vi "VP_AIT 1553 Get BM MonitorData Message At.vi"(7 "error in":errorcluster, 9 "message index in":u32, 10 "monitor data handle in":u32) -> (0 "error out":errorcluster, 2 "VP BM Message":T1[](array[typedef]) {"Data Word array" format="%x"}, 3 "monitor data handle out":u32)   [LabVIEW 2013]
doc: "Returns a summary cluster of the message at a given message index."
uses:
  RT Controls/VP_BM Message.ctl
  <instrlib>/AIT 1553/Private/AIT 1553 Utility/Decode Word/Decode Word (Command as terminals).vi
  <userlib>/MIL-STD-1553/Owl1553.lvlib
  AIT 664 Custom Device.lvlib
  <instrlib>/AIT 1553/AIT 1553.lvlib
panel:
  out "Message We Want":bool
  # "(c) 2010 Avionics Interface Technologies.  ALL RIGHTS RESERVED."
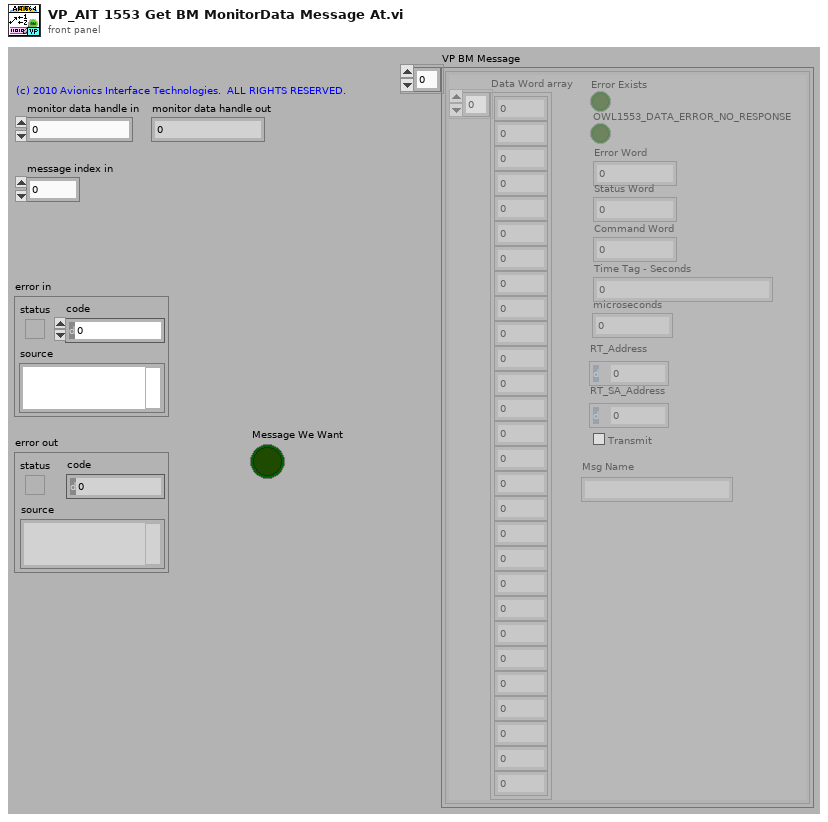
[diagram p1: front panel]
types:
  T1 = typedef "AIT 664 Custom Device.lvlib/VP_BM Message.ctl" = cluster{"Data Word array":u16[], "Error Exists":bool, "OWL1553_DATA_ERROR_NO_RESPONSE":bool, "Error Word":u32, "Status Word":u16, "Command Word":u16, "Time Tag - Seconds":u32, "microseconds":u32, "RT_Address":u8, "RT_SA_Address":u8, "Transmit":bool, "Msg Name":string}
  T2 = enum16{"BCRT", "RTBC", "RTRT", "FRONT_HALF", "BACK_HALF", "MSG_ERROR"}
  T3 = enum16{"OWL1553_BCRT", "OWL1553_RTBC", "OWL1553_RTRT", "OWL1553_FRONT_HALF", "OWL1553_BACK_HALF", "OWL1553_MSG_ERROR"}
  T4 = cluster{"day":u32, "hour":u32, "minute":u32, "second":u32, "microsecond":u32}
  T5 = cluster{"OWL1553_DATA_ERROR_ALTERNATE_BUS":bool, "OWL1553_DATA_ERROR_WORDCOUNT_LOW":bool, "OWL1553_DATA_ERROR_WORDCOUNT_HIGH":bool, "OWL1553_DATA_ERROR_STATUS_WORD":bool, "OWL1553_DATA_ERROR_TERMINAL_ADDRESS":bool, "OWL1553_DATA_ERROR_GAP_SHORT":bool, "OWL1553_DATA_ERROR_ILLEGAL_COMMAND":bool, "OWL1553_DATA_ERROR_BOTH_BUSES":bool, "OWL1553_DATA_ERROR_INTERWORD_GAP":bool, "OWL1553_DATA_ERROR_INVERTED_SYNC":bool, "OWL1553_DATA_ERROR_PARITY":bool, "OWL1553_DATA_ERROR_BITCOUNT_HIGH":bool, "OWL1553_DATA_ERROR_BITCOUNT_LOW":bool, "OWL1553_DATA_ERROR_MANCHESTER":bool, "OWL1553_DATA_ERROR_MANCHESTER_HIGH":bool, "OWL1553_DATA_ERROR_MANCHESTER_LOW":bool, "OWL1553_DATA_ERROR_NO_RESPONSE":bool, "OWL1553_DATA_ERROR_ZERO_CROSSING":bool}
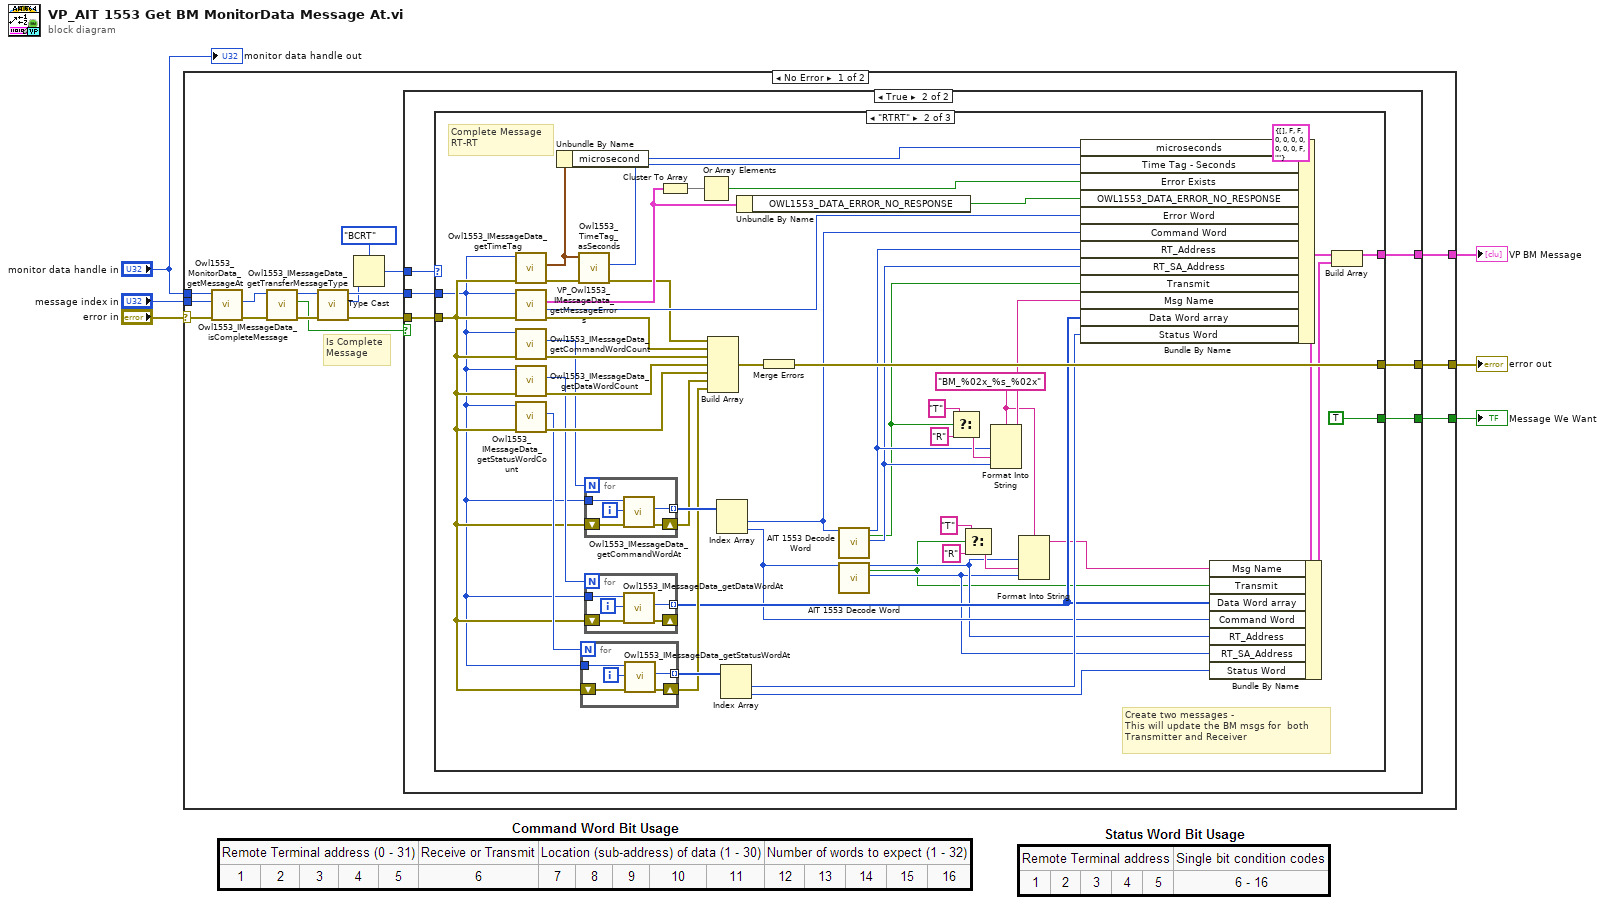
[diagram p0: block diagram]
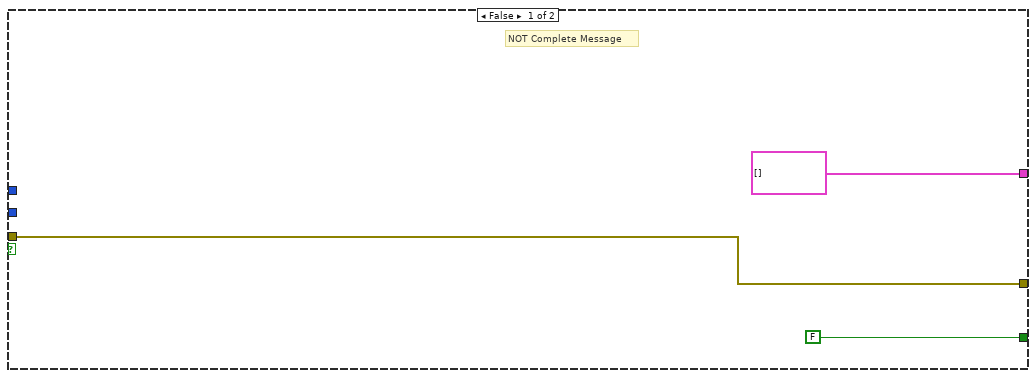
[diagram p2: hidden frame]
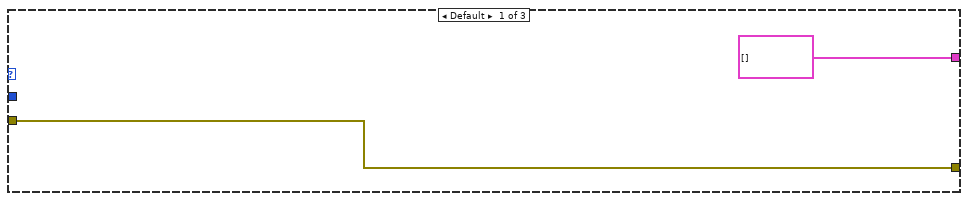
[diagram p3: hidden frame]
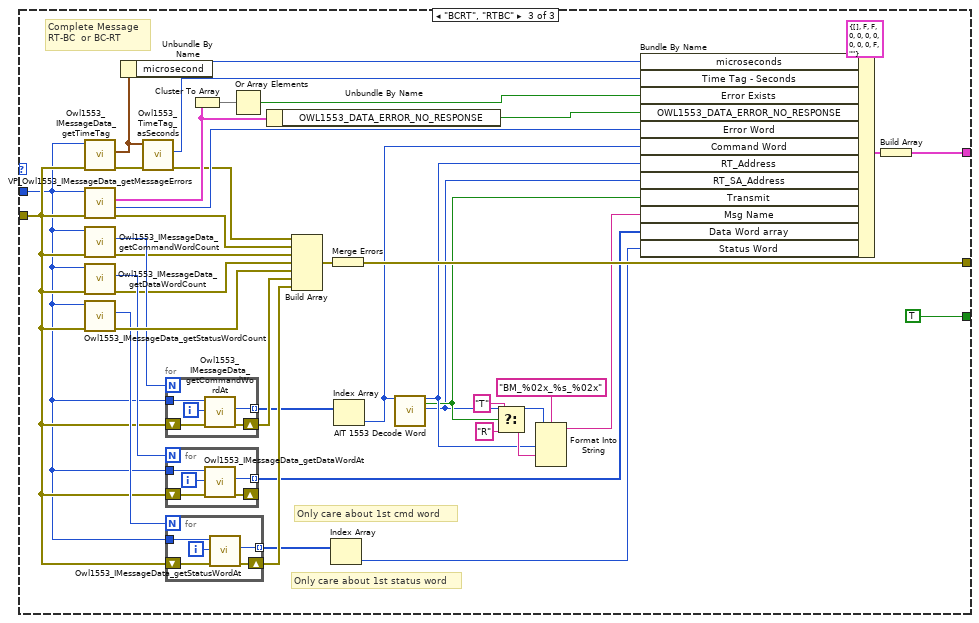
[diagram p4: hidden frame]
diagram:
  n1 = case shown="No Error" "error in" {
    selector: "error in" -> [w21 w154]
    tunnel: [w19 w154] -> w3
    tunnel: "monitor data handle in" -> [w18 _]
    tunnel: "message index in" -> [w22 _]
    tunnel: [w20 _] -> w1
    tunnel: [w9 _] -> w2
    frame No Error {
      # "Is Complete\nMessage"
      n2 = call <userlib>:"Owl1553_MonitorData_getMessageAt.vi"("error in (no error)"=w21, "index"=w22, "monitor data handle"=w18) -> ("error out"=w17:errorcluster, "imessage data handle"=w16:u64)  [unwired: 6 in, 1 out]
      n3 = call <userlib>:"Owl1553_IMessageData_isCompleteMessage.vi"("error in (no error)"=w17, "imessage data handle"=w16) -> ("error out"=w14:errorcluster, "complete"=w8:bool, "imessage data handle"=w15:u64)  [unwired: 7 in]
      n4 = call <userlib>:"Owl1553_IMessageData_getTransferMessageType.vi"("error in (no error)"=w14, "IMessageData handle"=w15) -> ("error out"=w13:errorcluster, "transferMessageType"=w11:T3, "IMessageData handle out"=w12:u64)  [unwired: 7 in]
      n5 = Type Cast(type=T2."BCRT" ("transfer type"), x=w11) -> (*(type *) &x=w7:T2)
      n6 = case shown="True" w8 {
        tunnel: [T1[] [] w31] -> w20
        tunnel: [w24 w30] -> w19
        tunnel: w13 -> [w24 w29]
        tunnel: w12 -> [_ w28]
        tunnel: [FALSE ("Message We Want") w27] -> w9
        tunnel: w7 -> [_ w26]
        frame False {
          # "NOT Complete Message"
        }
        frame True {
          n7 = case shown="\"RTRT\"" w26 {
            tunnel: [T1[] [] w65 w120] -> w31
            tunnel: [w33 w79 w136] -> w30
            tunnel: w29 -> [w33 w68 w123]
            tunnel: w28 -> [_ w67 w122]
            tunnel: [_ TRUE ("Message We Want") TRUE ("Message We Want")] -> w27
            frame Default {
            }
            frame "RTRT" {
              w40 = "BM_%02x_%s_%02x"
              # "Create two messages - \nThis will update the BM msgs for  both\nTransmitter and Receiver"
              # "Complete Message\nRT-RT"
              n8 = call <userlib>:"Owl1553_IMessageData_getTimeTag.vi"("error in (no error)"=w68, "imessage data handle"=w67) -> ("error out"=w74:errorcluster, "time tag"=w71:T4)  [unwired: 7 in, 1 out]
              n9 = call "VP_Owl1553_IMessageData_getMessageErrors.vi"("error in (no error)"=w68, "imessage data handle"=w67) -> ("error out"=w36:errorcluster, "error word"=w69:u32, "DataErrorType"=w57:T5)  [unwired: 6 in, 1 out]
              n10 = call <userlib>:"Owl1553_IMessageData_getCommandWordCount.vi"("error in (no error)"=w68, "imessage data handle"=w67) -> ("error out"=w83:errorcluster, "word count"=w76:u8)  [unwired: 7 in, 1 out]
              n11 = call <userlib>:"Owl1553_IMessageData_getDataWordCount.vi"("error in (no error)"=w68, "imessage data handle"=w67) -> ("error out"=w82:errorcluster, "word count"=w78:u8)  [unwired: 7 in, 1 out]
              n12 = call <userlib>:"Owl1553_IMessageData_getStatusWordCount.vi"("error in (no error)"=w68, "imessage data handle"=w67) -> ("error out"=w81:errorcluster, "word count"=w75:u8)  [unwired: 7 in, 1 out]
              n13 = Unbundle By Name(w71) -> ("microsecond"=w39:u32)
              n14 = call <userlib>:"Owl1553_TimeTag_asSeconds.vi"("error in (no error)"=w74, "time tag"=w71) -> ("error out"=w37:errorcluster, "seconds"=w38:u32)  [unwired: 7 in, 1 out]
              n15 = for {
                N: w75 -> [_]
                shift-right: [w91] -> w53
                shift-left: w68 -> [w92]
                tunnel: w67 -> [w90]
                tunnel: [w89] -> w59 mode=indexing
                i -> [w93]
                n16 = call <userlib>:"Owl1553_IMessageData_getStatusWordAt.vi"("error in (no error)"=w92, "status word index"=w93, "imessage data handle"=w90) -> ("error out"=w91:errorcluster, "word"=w89:u16)  [unwired: 6 in, 1 out]
              }
              n17 = for {
                N: w76 -> [_]
                shift-right: [w86] -> w56
                shift-left: w68 -> [w87]
                tunnel: w67 -> [w85]
                tunnel: [w84] -> w58 mode=indexing
                i -> [w88]
                n18 = call <userlib>:"Owl1553_IMessageData_getCommandWordAt.vi"("error in (no error)"=w87, "command word index"=w88, "imessage data handle"=w85) -> ("error out"=w86:errorcluster, "word"=w84:u16)  [unwired: 6 in, 1 out]
              }
              n19 = for {
                N: w78 -> [_]
                tunnel: w67 -> [w97]
                shift-right: [w94] -> _
                shift-left: w68 -> [w96]
                tunnel: [w95] -> w47 mode=indexing
                i -> [w98]
                n20 = call <userlib>:"Owl1553_IMessageData_getDataWordAt.vi"("error in (no error)"=w96, "data word index"=w98, "imessage data handle"=w97) -> ("error out"=w94:errorcluster, "word"=w95:u16)  [unwired: 6 in, 1 out]
              }
              n21 = Cluster To Array(cluster=w57) -> (array=w77:bool[])
              n22 = Or Array Elements(Boolean array=w77) -> (logical OR=w72:bool)
              n23 = Build Array(w37, w36, w83, w82, w81, w56, w53) -> (w80:errorcluster[])
              n24 = Index Array(array=w58) -> (element #1=w35:u16, element #2=w45:u16)  [unwired: 2 in]
              n25 = Index Array(array=w59) -> (element #1=w54:u16, element #2=w46:u16)  [unwired: 2 in]
              n26 = Unbundle By Name(w57) -> ("OWL1553_DATA_ERROR_NO_RESPONSE"=w70:bool)
              n27 = Merge Errors(w80) -> (w79:errorcluster)
              n28 = call-poly <instrlib>:"AIT 1553 Decode Word.vi"("command word in"=w35) -> ("remote terminal address out"=w61:u16, "transmit out"=w49:bool, "subaddress / mode out"=w60:u16)  [unwired: 15 in, 1 out]
              n29 = call-poly <instrlib>:"AIT 1553 Decode Word.vi"("command word in"=w45) -> ("remote terminal address out"=w44:u16, "transmit out"=w42:bool, "subaddress / mode out"=w43:u16)  [unwired: 15 in, 1 out]
              n30 = Select(t="T", s=w49, f="R") -> (s? t:f=w62:string)
              n31 = Select(t="T", s=w42, f="R") -> (s? t:f=w52:string)
              n32 = Format Into String(format string=w40, w61, w62, w60) -> (resulting string=w55:string)  [unwired: 2 in, 1 out]
              n33 = Format Into String(format string=w40, w44, w52, w43) -> (resulting string=w34:string)  [unwired: 2 in, 1 out]
              n34 = Bundle By Name(cluster=T1 {"Data Word array"=[], "Error Exists"=FALSE, "OWL1553_DATA_ERROR_NO_RESPONSE"=FALSE, "Error Word"=0, "Status Word"=0, "Command Word"=0, "Time Tag - Seconds"=0, "microseconds"=0, "RT_Address"=0, "RT_SA_Address"=0, "Transmit"=FALSE, "Msg Name"=""} ("VP BM Message"), "microseconds"=w39, "Time Tag - Seconds"=w38, "Error Exists"=w72, "OWL1553_DATA_ERROR_NO_RESPONSE"=w70, "Error Word"=w69, "Command Word"=w35, "RT_Address"=w61, "RT_SA_Address"=w60, "Transmit"=w49, "Msg Name"=w55, "Data Word array"=w47, "Status Word"=w54) -> (w48:T1)
              n35 = Bundle By Name(cluster=w48, "Msg Name"=w34, "Transmit"=w42, "Data Word array"=w47, "Command Word"=w45, "RT_Address"=w44, "RT_SA_Address"=w43, "Status Word"=w46) -> (w41:T1)
              n36 = Build Array(w48, w41) -> (w65:T1[])
            }
            frame "BCRT", "RTBC" {
              # "Only care about 1st cmd word"
              # "Only care about 1st status word"
              # "Complete Message\nRT-BC  or BC-RT"
              n37 = call <userlib>:"Owl1553_IMessageData_getTimeTag.vi"("error in (no error)"=w123, "imessage data handle"=w122) -> ("error out"=w129:errorcluster, "time tag"=w126:T4)  [unwired: 7 in, 1 out]
              n38 = call "VP_Owl1553_IMessageData_getMessageErrors.vi"("error in (no error)"=w123, "imessage data handle"=w122) -> ("error out"=w101:errorcluster, "error word"=w104:u32, "DataErrorType"=w125:T5)  [unwired: 6 in, 1 out]
              n39 = call <userlib>:"Owl1553_IMessageData_getCommandWordCount.vi"("error in (no error)"=w123, "imessage data handle"=w122) -> ("error out"=w110:errorcluster, "word count"=w131:u8)  [unwired: 7 in, 1 out]
              n40 = call <userlib>:"Owl1553_IMessageData_getDataWordCount.vi"("error in (no error)"=w123, "imessage data handle"=w122) -> ("error out"=w109:errorcluster, "word count"=w135:u8)  [unwired: 7 in, 1 out]
              n41 = call <userlib>:"Owl1553_IMessageData_getStatusWordCount.vi"("error in (no error)"=w123, "imessage data handle"=w122) -> ("error out"=w138:errorcluster, "word count"=w130:u8)  [unwired: 7 in, 1 out]
              n42 = Unbundle By Name(w126) -> ("microsecond"=w106:u32)
              n43 = call <userlib>:"Owl1553_TimeTag_asSeconds.vi"("error in (no error)"=w129, "time tag"=w126) -> ("error out"=w102:errorcluster, "seconds"=w105:u32)  [unwired: 7 in, 1 out]
              n44 = for {
                N: w131 -> [_]
                shift-right: [w141] -> w133
                shift-left: w123 -> [w142]
                tunnel: w122 -> [w140]
                tunnel: [w139] -> w111 mode=indexing
                i -> [w143]
                n45 = call <userlib>:"Owl1553_IMessageData_getCommandWordAt.vi"("error in (no error)"=w142, "command word index"=w143, "imessage data handle"=w140) -> ("error out"=w141:errorcluster, "word"=w139:u16)  [unwired: 6 in, 1 out]
              }
              n46 = for {
                N: w135 -> [_]
                tunnel: w122 -> [w152]
                shift-right: [w149] -> _
                shift-left: w123 -> [w151]
                tunnel: [w150] -> w107 mode=indexing
                i -> [w153]
                n47 = call <userlib>:"Owl1553_IMessageData_getDataWordAt.vi"("error in (no error)"=w151, "data word index"=w153, "imessage data handle"=w152) -> ("error out"=w149:errorcluster, "word"=w150:u16)  [unwired: 6 in, 1 out]
              }
              n48 = for {
                N: w130 -> [_]
                shift-right: [w146] -> w132
                shift-left: w123 -> [w147]
                tunnel: w122 -> [w145]
                tunnel: [w144] -> w112 mode=indexing
                i -> [w148]
                n49 = call <userlib>:"Owl1553_IMessageData_getStatusWordAt.vi"("error in (no error)"=w147, "status word index"=w148, "imessage data handle"=w145) -> ("error out"=w146:errorcluster, "word"=w144:u16)  [unwired: 6 in, 1 out]
              }
              n50 = Cluster To Array(cluster=w125) -> (array=w134:bool[])
              n51 = Or Array Elements(Boolean array=w134) -> (logical OR=w127:bool)
              n52 = Unbundle By Name(w125) -> ("OWL1553_DATA_ERROR_NO_RESPONSE"=w124:bool)
              n53 = Build Array(w102, w101, w110, w109, w138, w133, w132) -> (w137:errorcluster[])
              n54 = Index Array(array=w112) -> (element=w103:u16)  [unwired: 1 in]
              n55 = Merge Errors(w137) -> (w136:errorcluster)
              n56 = Index Array(array=w111) -> (element=w100:u16)  [unwired: 1 in]
              n57 = call-poly <instrlib>:"AIT 1553 Decode Word.vi"("command word in"=w100) -> ("remote terminal address out"=w115:u16, "transmit out"=w114:bool, "subaddress / mode out"=w113:u16)  [unwired: 15 in, 1 out]
              n58 = Select(t="T", s=w114, f="R") -> (s? t:f=w116:string)
              n59 = Format Into String(format string="BM_%02x_%s_%02x", w115, w116, w113) -> (resulting string=w108:string)  [unwired: 2 in, 1 out]
              n60 = Bundle By Name(cluster=T1 {"Data Word array"=[], "Error Exists"=FALSE, "OWL1553_DATA_ERROR_NO_RESPONSE"=FALSE, "Error Word"=0, "Status Word"=0, "Command Word"=0, "Time Tag - Seconds"=0, "microseconds"=0, "RT_Address"=0, "RT_SA_Address"=0, "Transmit"=FALSE, "Msg Name"=""} ("VP BM Message"), "microseconds"=w106, "Time Tag - Seconds"=w105, "Error Exists"=w127, "OWL1553_DATA_ERROR_NO_RESPONSE"=w124, "Error Word"=w104, "Command Word"=w100, "RT_Address"=w115, "RT_SA_Address"=w113, "Transmit"=w114, "Msg Name"=w108, "Data Word array"=w107, "Status Word"=w103) -> (w99:T1)
              n61 = Build Array(w99) -> (w120:T1[])
            }
          }
        }
      }
    }
    frame Error {
    }
  }
  "error out" <- w3
  "Message We Want" <- w2
  "VP BM Message" <- w1
  "monitor data handle out" <- "monitor data handle in"
